vi "EMBL 4Pi Shutter Engine.vi"(0 "Unique Notifier Name":string="Not a Name", 11 "COM Port":string[](array[string])) -> ()   [LabVIEW 2020]
uses:
  Shutter Controls/Shutter Notifier Element.ctl
  Shutter Controls/Shutter Actions.ctl
  <vilib>/Instr/_visa.llb/VISA Configure Serial Port (Instr).vi
panel:
  in  "Quit":bool
  in  "Shutter":bool
  # "1: Com Port\n2: Close Command\n3: Open Command"
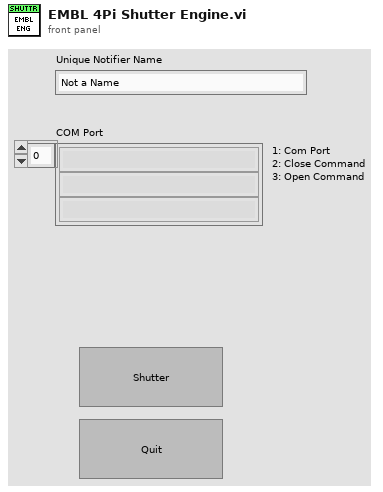
[diagram p1: front panel]
types:
  T1 = typedef "Shutter Notifier Element.ctl" = cluster{"Action":T2, "Status":T2, "Received?":bool}
  T2 = typedef "Shutter Actions.ctl" = enum16{"Open", "Close", "Toggle", "Status", "Quit"}
  T3 = enum32{"Invalid", "Standard", "Closed", "Hidden", "Minimized", "Maximized"}
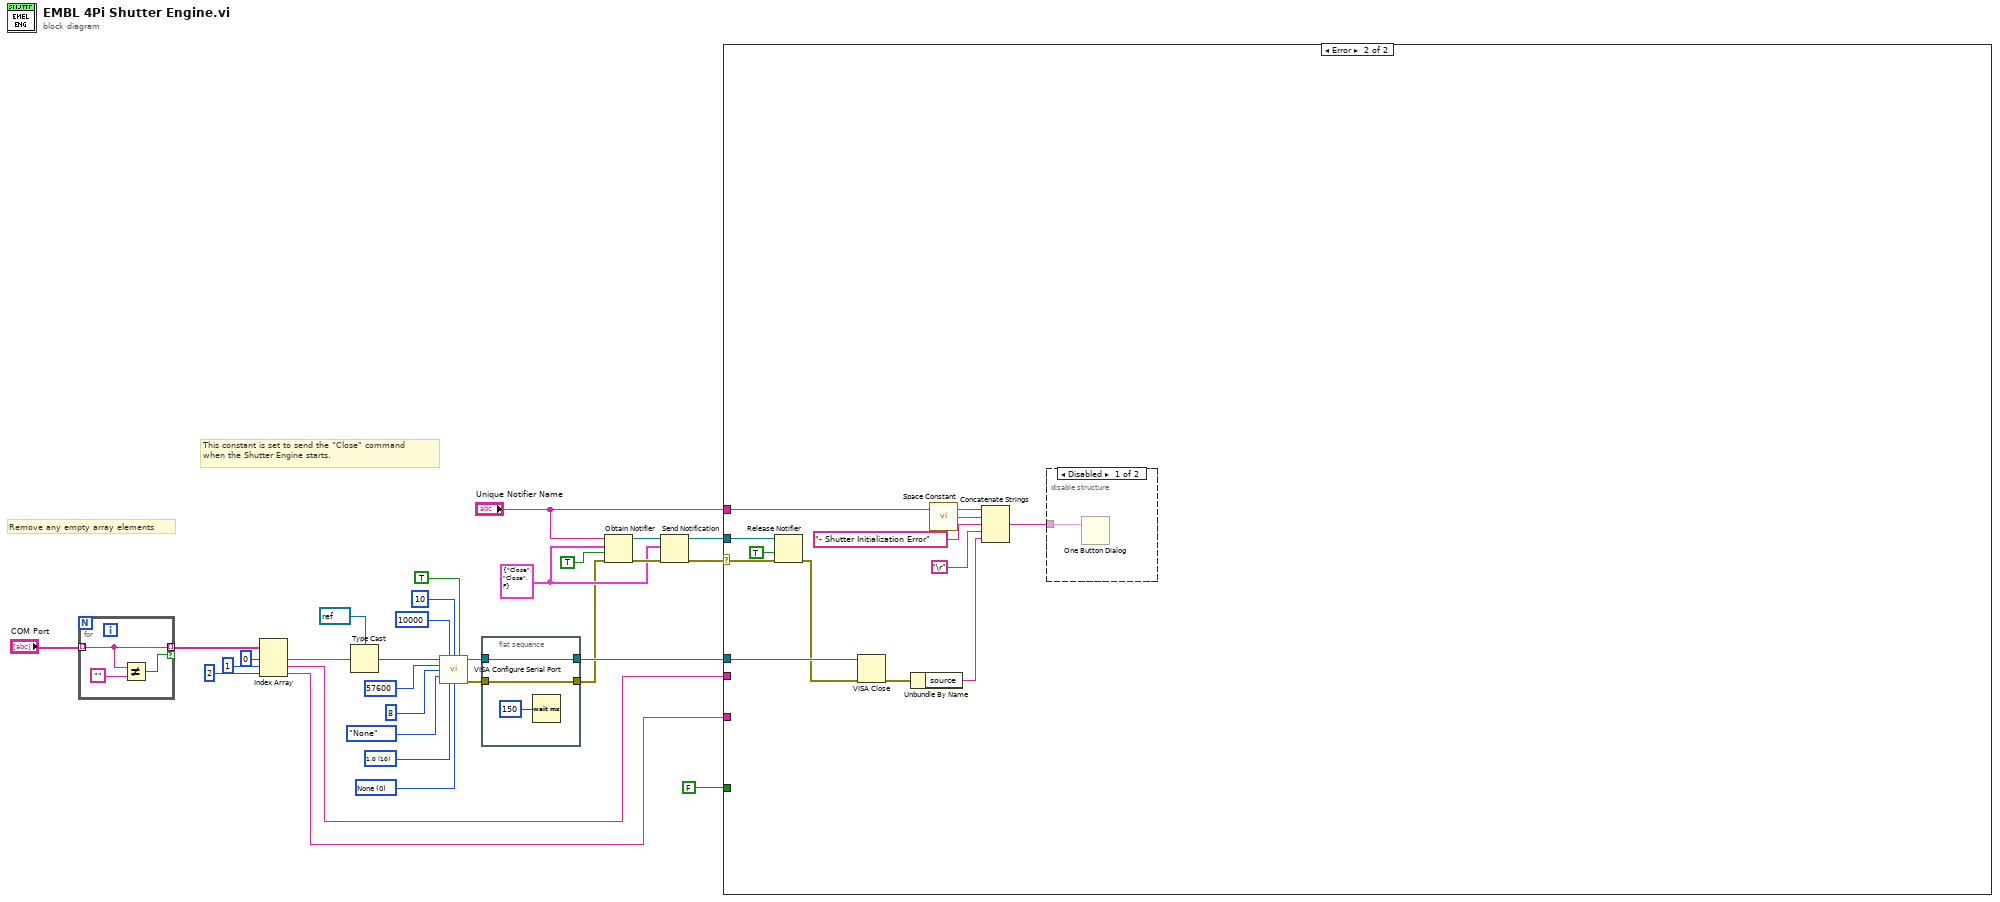
[diagram p0: block diagram]
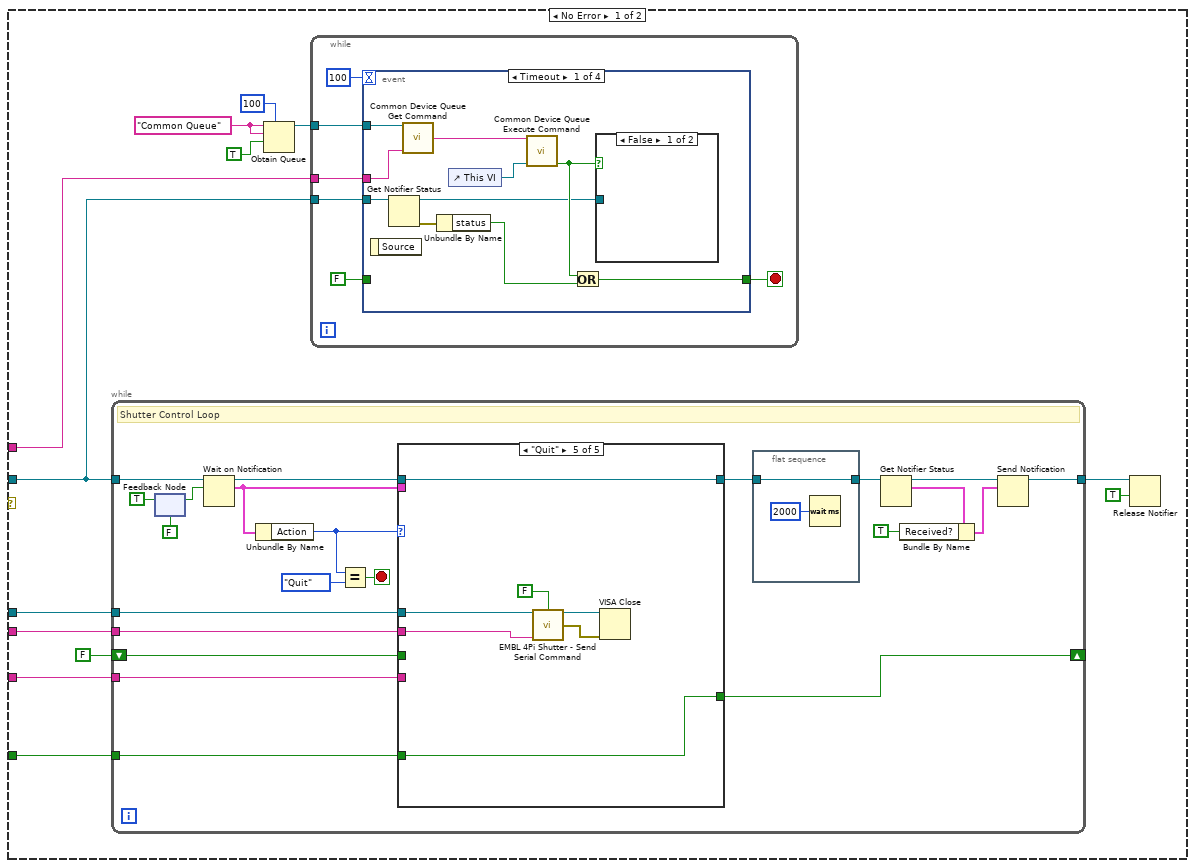
[diagram p2: hidden frame]
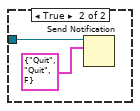
[diagram p3: hidden frame]
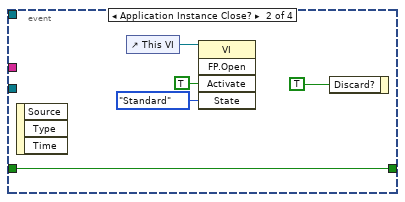
[diagram p4: hidden frame]
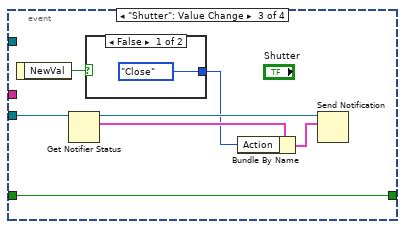
[diagram p5: hidden frame]
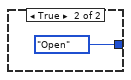
[diagram p6: hidden frame]
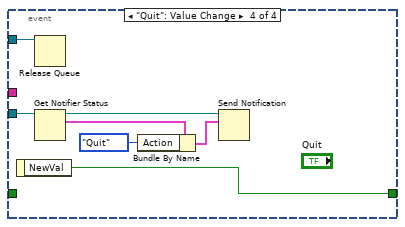
[diagram p7: hidden frame]
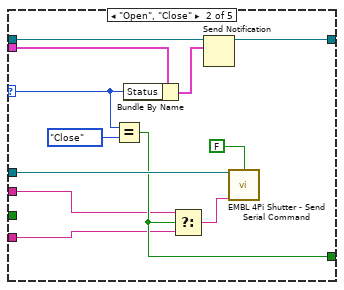
[diagram p9: hidden frame]
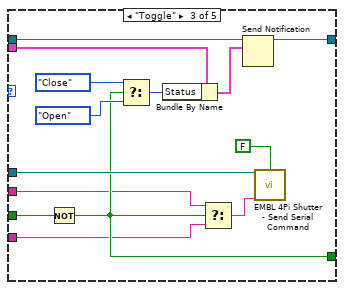
[diagram p10: hidden frame]
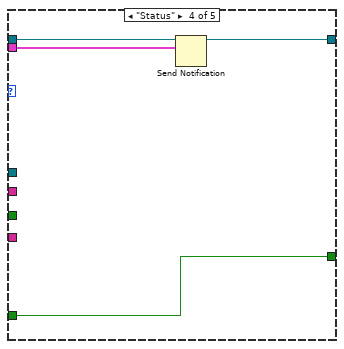
[diagram p11: hidden frame]
diagram:
  w16 = u16 0 items=["None", "XON/XOFF", "RTS/CTS", "XON/XOFF & RTS/CTS", "DTR/DSR", "XON/XOFF & DTR/DSR"] ("flow control (0:none)")
  w17 = u16 10 items=["1.0"=10, "1.5"=15, "2.0"=20] ("stop bits (10: 1 bit)")
  w26 = T1 {"Action"=enum."Close", "Status"=enum."Close", "Received?"=FALSE} ("Shutter Notifier Element")
  # "Remove any empty array elements"
  # "This constant is set to send the \"Close\" command\nwhen the Shutter Engine starts."
  n1 = for {
    tunnel: "COM Port" -> [w32] mode=indexing
    tunnel: [w32] -> w13 mode=indexing if=w31
    n2 = Not Equal?(x=w32, y="") -> (x != y?=w31:bool)
  }
  n3 = Index Array(array=w13, index #1=0 ("index"), index #2=1 ("index"), index #3=2 ("index")) -> (element #1=w11:string, element #2=w5:string, element #3=w6:string)
  n4 = Type Cast(type=refnum<visa-resource-name> refnum ("reference out"), x=w11) -> (*(type *) &x=w10:refnum<visa-resource-name>)
  n5 = call-poly "VISA Configure Serial Port"("VISA resource name"=w10, "timeout (10sec)"=u32 10000, "termination char\n(0xA = '\\n' = LF)"=u8 10 ("termination char\n(0xA = '\\n' = LF)"), "Enable Termination\nChar (T)"=TRUE ("Enable Termination\nChar (T)"), "baud rate (9600)"=u32 57600, "data bits (8)"=u16 8, "parity (0:none)"=enum16{"None", "Odd", "Even", "Mark", "Space"}."None", "stop bits (10: 1 bit)"=w17, "flow control (0:none)"=w16) -> ("VISA resource name out"=w4:refnum<visa-resource-name>, "error out"=w2:errorcluster)  [unwired: 5 in]
  n6 = flat-sequence {
    tunnel: w4 -> [w36]
    tunnel: [w36] -> w3
    tunnel: [w35] -> w1
    tunnel: w2 -> [w35]
    frame #0 {
      n7 = Wait (ms)(milliseconds to wait=u32 150) -> ()  [unwired: 1 out]
    }
  }
  n8 = Obtain Notifier(name (unnamed)="Unique Notifier Name", notification data type=w26, create if not found? (T)=TRUE, error in (no error)=w1) -> (notifier out=w29:refnum<notifier>, error out=w28:errorcluster)  [unwired: 1 out]
  n9 = Send Notification(notification=w26, notifier=w29, error in (no error)=w28) -> (notifier out=w27:refnum<notifier>, error out=w25:errorcluster)
  n10 = case shown="Error" w25 {
    selector: w25 -> [_ w161]
    tunnel: w3 -> [w49 w154]
    tunnel: w27 -> [w45 w162]
    tunnel: "Unique Notifier Name" -> [w44 w160]
    tunnel: FALSE -> [w46 _]
    tunnel: w6 -> [w38 _]
    tunnel: w5 -> [w37 _]
    frame No Error {
      w42 = "Common Queue" ("Unique Notifier Name")
      n11 = while {
        tunnel: w45 -> [w102]
        tunnel: w49 -> [w108]
        tunnel: [w103] -> w47
        tunnel: w46 -> [w95]
        shift-right: [w93] -> _
        shift-left: FALSE -> [w94]
        tunnel: w38 -> [w92]
        tunnel: w37 -> [w91]
        stop <- w109 stop-if-true
        # "Shutter Control Loop"
        n12 = feedback #1(FALSE) -> (w98:bool)
        n13 = feedback-in #1(TRUE) -> ()
        n14 = Wait on Notification(notifier=w102, ignore previous (F)=w98) -> (notifier out=w101:refnum<notifier>, notification=w97:T1)  [unwired: 2 in, 2 out]
        n15 = Unbundle By Name(w97) -> ("Action"=w96:T2)
        n16 = Equal?(x=w96, y=Shutter_Actions."Quit") -> (x = y?=w109:bool)
        n17 = case shown="\"Quit\"" w96 {
          selector: w96 -> [_ w121 _ _ _]
          tunnel: w101 -> [w114 w124 w138 w143 w151]
          tunnel: w108 -> [_ w120 w131 _ w149]
          tunnel: [w114 w125 w137 w144 w151] -> w90
          tunnel: w97 -> [_ w123 w136 w142 _]
          tunnel: w95 -> [_ _ _ w141 w150]
          tunnel: w94 -> [w113 _ w140 _ _]
          tunnel: [w113 w119 w130 w141 w150] -> w93
          tunnel: w92 -> [_ w115 w128 _ _]
          tunnel: w91 -> [_ w116 w127 _ w145]
          frame Default {
          }
          frame "Open", "Close" {
            n18 = Equal?(x=w121, y=Shutter_Actions."Close") -> (x = y?=w119:bool)
            n19 = Bundle By Name(cluster=w123, "Status"=w121) -> (w126:T1)
            n20 = Select(t=w116, s=w119, f=w115) -> (s? t:f=w118:string)
            n21 = Send Notification(notification=w126, notifier=w124) -> (notifier out=w125:refnum<notifier>)  [unwired: 1 in, 1 out]
            n22 = call "EMBL 4Pi Shutter - Send Serial Command.vi"("VISA Ref"=w120, "Wait for Reply?"=FALSE, "Command"=w118) -> ()  [unwired: 10 in, 3 out]
          }
          frame "Toggle" {
            n23 = Not(x=w140) -> (.not. x?=w130:bool)
            n24 = Select(t=Shutter_Actions."Close" ("Status"), s=w130, f=Shutter_Actions."Open" ("Status")) -> (s? t:f=w133:T2)
            n25 = Bundle By Name(cluster=w136, "Status"=w133) -> (w139:T1)
            n26 = Select(t=w127, s=w130, f=w128) -> (s? t:f=w132:string)
            n27 = Send Notification(notification=w139, notifier=w138) -> (notifier out=w137:refnum<notifier>)  [unwired: 1 in, 1 out]
            n28 = call "EMBL 4Pi Shutter - Send Serial Command.vi"("VISA Ref"=w131, "Wait for Reply?"=FALSE, "Command"=w132) -> ()  [unwired: 10 in, 3 out]
          }
          frame "Status" {
            n29 = Send Notification(notification=w142, notifier=w143) -> (notifier out=w144:refnum<notifier>)  [unwired: 1 in, 1 out]
          }
          frame "Quit" {
            n30 = call "EMBL 4Pi Shutter - Send Serial Command.vi"("VISA Ref"=w149, "Wait for Reply?"=FALSE, "Command"=w145) -> ("VISA Ref Out"=w148:refnum<visa-resource-name>, "Error Out"=w146:errorcluster)  [unwired: 10 in, 1 out]
            n31 = VISA Close(VISA resource name=w148, error in (no error)=w146) -> ()  [unwired: 1 out]
          }
        }
        n32 = flat-sequence {
          tunnel: w90 -> [w112]
          tunnel: [w112] -> w89
          frame #0 {
            n33 = Wait (ms)(milliseconds to wait=u32 2000) -> ()  [unwired: 1 out]
          }
        }
        n34 = Get Notifier Status(notifier=w89) -> (notifier out=w104:refnum<notifier>, current notification=w106:T1)  [unwired: 1 in, 3 out]
        n35 = Bundle By Name(cluster=w106, "Received?"=TRUE) -> (w107:T1)
        n36 = Send Notification(notification=w107, notifier=w104) -> (notifier out=w103:refnum<notifier>)  [unwired: 1 in, 1 out]
      }
      n37 = Obtain Queue(max queue size (-1, unlimited)=100, name (unnamed)=w42, element data type=w42, create if not found? (T)=TRUE) -> (queue out=w39:refnum<queue>)  [unwired: 1 in, 2 out]
      n38 = while {
        tunnel: w39 -> [w55]
        tunnel: w45 -> [w52]
        tunnel: w44 -> [w50]
        stop <- w51 stop-if-true
        n39 = event shown="[0] Timeout" {
          selector: _ -> [_ _ _ _]
          dyn-events: _ -> [_ _ _ _]
          timeout: 100 -> [_ _ _ _]
          tunnel: w55 -> [w63 _ _ w82]
          tunnel: FALSE -> [_ w72 w75 _]
          tunnel: w52 -> [w65 _ w79 w83]
          tunnel: [w58 w72 w75 w88] -> w51
          tunnel: w50 -> [w62 _ _ _]
          event Timeout {
            n40 = event-data() -> ()  [unwired: 1 in, 1 out]
            n41 = Get Notifier Status(notifier=w65) -> (notifier out=w56:refnum<notifier>, error out=w64:errorcluster)  [unwired: 1 in, 3 out]
            n42 = call "Common Device Queue Get Command.vi"("Common Queue"=w63, "Notifier Name"=w62) -> ("Command"=w61:string)  [unwired: 12 in, 1 out]
            n43 = Unbundle By Name(w64) -> ("status"=w59:bool)
            n44 = control-ref of="This VI"() -> (w60:refnum<vi>)
            n45 = call "Common Device Queue Execute Command.vi"("Common Command"=w61, "VI Refnum"=w60) -> ("Quit?"=w57:bool)  [unwired: 12 in, 1 out]
            n46 = Or(x=w57, y=w59) -> (x .or. y?=w58:bool)
            n47 = case shown="False" w57 {
              tunnel: w56 -> [_ w67]
              frame False {
              }
              frame True {
                n48 = Send Notification(notification=T1 {"Action"=enum."Quit", "Status"=enum."Quit", "Received?"=FALSE} ("Shutter Notifier Element"), notifier=w67) -> ()  [unwired: 1 in, 2 out]
              }
            }
          }
          event Application Instance Close? {
            n49 = event-data() -> ()  [unwired: 1 in, 3 out]
            n50 = control-ref of="This VI"() -> (w69:refnum<vi>)
            n51 = invoke class="VI" method="FP.Open"(reference=w69, "Activate"=TRUE ("Activate?"), "State"=T3."Standard") -> ()  [unwired: 2 in, 5 out]
            n52 = event-data("Discard?"=TRUE) -> ()  [unwired: 1 in, 1 out]
          }
          event "Shutter": Value Change {
            n53 = event-data() -> ("NewVal"=w74:bool)  [unwired: 1 in]
            n54 = Get Notifier Status(notifier=w79) -> (notifier out=w78:refnum<notifier>, current notification=w77:T1)  [unwired: 1 in, 3 out]
            n55 = case shown="False" w74 {
              tunnel: [Shutter_Actions."Close" ("Action") Shutter_Actions."Open" ("Action")] -> w73
              frame False {
              }
              frame True {
              }
            }
            n56 = Bundle By Name(cluster=w77, "Action"=w73) -> (w76:T1)
            n57 = Send Notification(notification=w76, notifier=w78) -> ()  [unwired: 1 in, 2 out]
          }
          event "Quit": Value Change {
            n58 = event-data() -> ("NewVal"=w88:bool)  [unwired: 1 in]
            n59 = Release Queue(queue=w82) -> ()  [unwired: 2 in, 3 out]
            n60 = Get Notifier Status(notifier=w83) -> (notifier out=w87:refnum<notifier>, current notification=w86:T1)  [unwired: 1 in, 3 out]
            n61 = Bundle By Name(cluster=w86, "Action"=Shutter_Actions."Quit") -> (w85:T1)
            n62 = Send Notification(notification=w85, notifier=w87) -> ()  [unwired: 1 in, 2 out]
          }
        }
      }
      n63 = Release Notifier(notifier=w47, force destroy? (F)=TRUE) -> ()  [unwired: 1 in, 3 out]
    }
    frame Error {
      n64 = Release Notifier(notifier=w162, force destroy? (F)=TRUE, error in (no error)=w161) -> (error out=w153:errorcluster)  [unwired: 2 out]
      n65 = VISA Close(VISA resource name=w154, error in (no error)=w153) -> (error out=w152:errorcluster)
      n66 = Unbundle By Name(w152) -> ("source"=w155:string)
      n67 = call <vilib>:"Space Constant.vi"() -> ("String"=w158:string)
      n68 = Concatenate Strings(w160, w158, "- Shutter Initialization Error" ("string"), "\r", w155) -> (w159:string)
      n69 = disable-structure shown="Disabled" {
        disable-tunnel: w159 -> [w164 _]
        frame Disabled {
          n70 = One Button Dialog(message=w164) -> ()  [unwired: 1 in, 1 out]
        }
        frame Enabled {
        }
      }
    }
  }
